vi "Write Subdiagram Label Target.vi"   [LabVIEW 2018, in "Toolkit.lvlib" / "Tests.lvlib"]
uses:
  Tests.lvlib
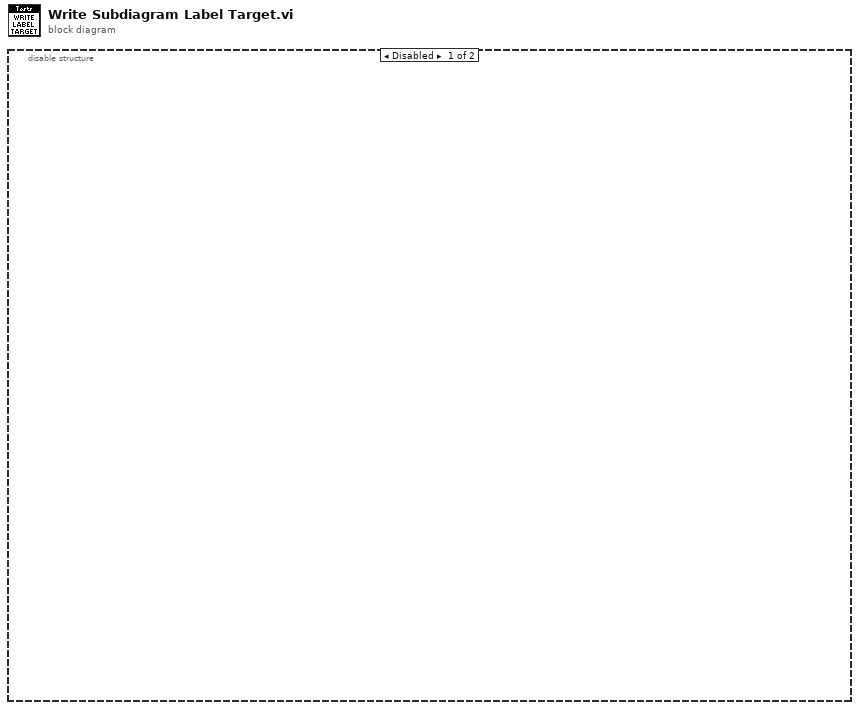
[diagram p0: block diagram]
diagram:
  n1 = disable-structure shown="Disabled" {
    frame Disabled {
    }
    frame Enabled {
    }
  }
